vi "Ribbon Page.vi"() -> ()   [LabVIEW 2020, in "3D Ribbon.lvclass"]
uses:
  <vilib>/Math Plots/3D Math Plots/3D Ribbon/3D Ribbon/3D Ribbon.lvclass
  <vilib>/Math Plots/3D Math Plots/3D Ribbon/3D Ribbon/Typedef/3D Ribbon Property Array.ctl
  <vilib>/Math Plots/3D Math Plots/3D Ribbon/3D Ribbon/Typedef/3D Ribbon Property.ctl
  <vilib>/Math Plots/3D Math Plots/3D Plot/3D Plot/Typedef/Color Ramp Cluster.ctl
  <vilib>/Math Plots/3D Math Plots/3D Plot/3D Plot/Typedef/Line Type.ctl
  <vilib>/Math Plots/3D Math Plots/3D Plot/3D Plot/Typedef/Dialog State.ctl
  <vilib>/Math Plots/3D Math Plots/3D Plot/3D Plot/Typedef/Temp Scene State.ctl
  <vilib>/Math Plots/3D Math Plots/3D Plot/3D Plot/Typedef/Temp Scene Property Action.ctl
  <vilib>/Math Plots/3D Math Plots/3D Plot/3D Plot/3D Plot.lvclass
panel:
  in  "Ribbon Width":sgl=0.001 caption="Ribbon width" min=0.001 max=10 step=0.1
  in  "Ribbon Mode":u16(ring) caption="Ribbon mode" items=["Row", "Column"]
  in  "Draw Ribbon":bool caption="Draw ribbon"
  in  "Line Style":u16(ring) caption="Line style"
  in  "Antialiasing":bool
  in  "Line Width":sgl caption="Line width" min=0.001 step=1
  in  "Line Color":u32(colorbox) caption="Line color"
  out "Ribbon Property Out":T1
  in  "Ribbon Property In":T1
  out "Color Ramp":dbl[][](graph)
  in  "Color Map Style":u16(ring) caption="Color map style" items=["None ", "Shaded", "Color spectrum", "Grey scale", "Custom"]
  in  "YZ Plane Projection":bool caption="YZ  plane projection"
  in  "XZ Plane Projection":bool caption="XZ  plane projection"
  in  "XY Plane Projection":bool caption="XY plane projection"
  in  "Coordinate System":u16(ring) caption="Coordinate system" items=["Cartesian", "Cylindrical", "Spherical"]
  in  "Plot Opacity":sgl(slide) caption="Plot opacity(%)" min=0 max=100 scale=0.0..100.0
  in  "Plot List":i32(listbox)
  in  "Ramp Edit":bool caption="Ramp edit"
  in  "Move Down":bool
  in  "Move Up":bool
  in  "Delete":bool
  in  "New":bool
  in  "Event Registration":refnum<event-registration>
  # "Ribbon"
  # "General"
  # "Projection"
  # "Color Ramp"
  # "Ribbon"
  # "Outline"
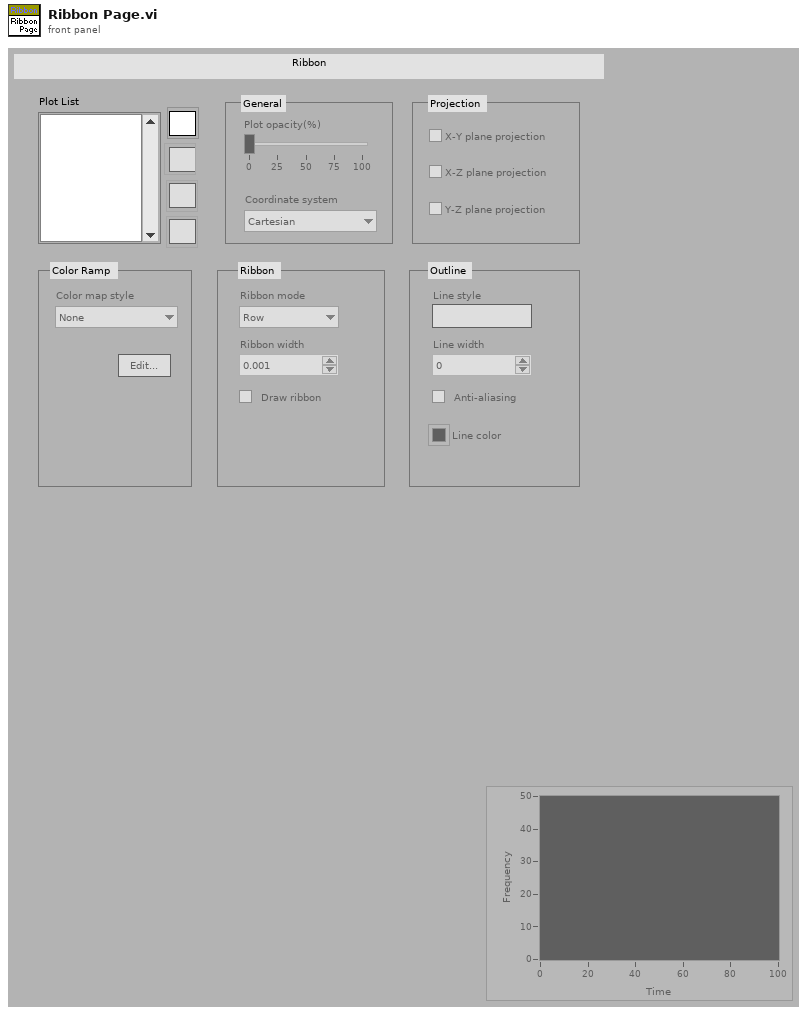
[diagram p1: front panel]
types:
  T1 = typedef "3D Ribbon.lvclass/3D Ribbon Property Array.ctl" = T2[]
  T2 = typedef "3D Ribbon.lvclass/3D Ribbon Property.ctl" = cluster{"General Property":cluster{"Plot Name":string, "Coordinate System":enum16{"Cartesian", "Cylindrical", "Spherical"}, "Opacity":sgl}, "Projection Property":cluster{"Draw XY":bool, "Draw YZ":bool, "Draw XZ":bool}, "Plot Property":cluster{"Draw Surface":bool, "Color Ramp Cluster":T3, "Line Style":T4, "Line Width":sgl, "Line Color":u32, "Antialiasing":bool}, "Ribbon Property":cluster{"Ribbon Mode":enum16{"Row", "Column"}, "Ribbon Width":sgl}}
  T3 = typedef "3D Plot.lvclass/Color Ramp Cluster.ctl" = cluster{"Color Ramp Style":enum16{"None", "Shaded", "Color spectrum", "Grey scale", "Custom"}, "Color Ramp Array":u32[], "Color Ramp Index":i32[], "Interpolate?":bool, "Logarithm?":bool}
  T4 = typedef "3D Plot.lvclass/Line Type.ctl" = enum16{"None", "Solid", "Dash", "Dot", "Dash Dot"}
  T5 = typedef "3D Plot.lvclass/Dialog State.ctl" = enum16{"Initialize", "Read Porperty", "Write Property", "Idle", "Exit"}
  T6 = typedef "3D Plot.lvclass/Temp Scene State.ctl" = enum16{"Create", "Update Scene", "Get Plot Representation", "Destory"}
  T7 = typedef "3D Plot.lvclass/Temp Scene Property Action.ctl" = enum16{"Graph Property", "Light Property", "Axis Property", "Value Pair Property", "Format Property", "Cursor Property", "Plot Specific Property"}
  T8 = typedef "3D Plot.lvclass/Multiplot Representation.ctl" = cluster{"Plot Represention Array":T9[], "Max Range":T10}
  T9 = typedef "3D Plot.lvclass/Plot Representation.ctl" = cluster{"Plot ID":i32, "Plot Range":T10, "Mesh Data":T11, "Dimension":cluster{"X Dimension":i32, "Y Dimension":i32}, "Ramp Range":T10}
  T10 = typedef "3D Plot.lvclass/Range Clusters.ctl" = cluster{"X Range":cluster{"Max X":sgl, "Min X":sgl}, "Y Range":cluster{"Max Y":sgl, "Min Y":sgl}, "Z Range":cluster{"Max Z":sgl, "Min Z":sgl}}
  T11 = typedef "3D Plot.lvclass/Mesh Data.ctl" = cluster{"Index Array":u32[], "Vertex Array":cluster{"X":sgl, "Y":sgl, "Z":sgl}[], "Normal Array":cluster{"X":sgl, "Y":sgl, "Z":sgl}[], "Color Index Array":i32[]}
  T12 = enum16{"None", "Shaded", "Color spectrum", "Grey scale", "Custom"}
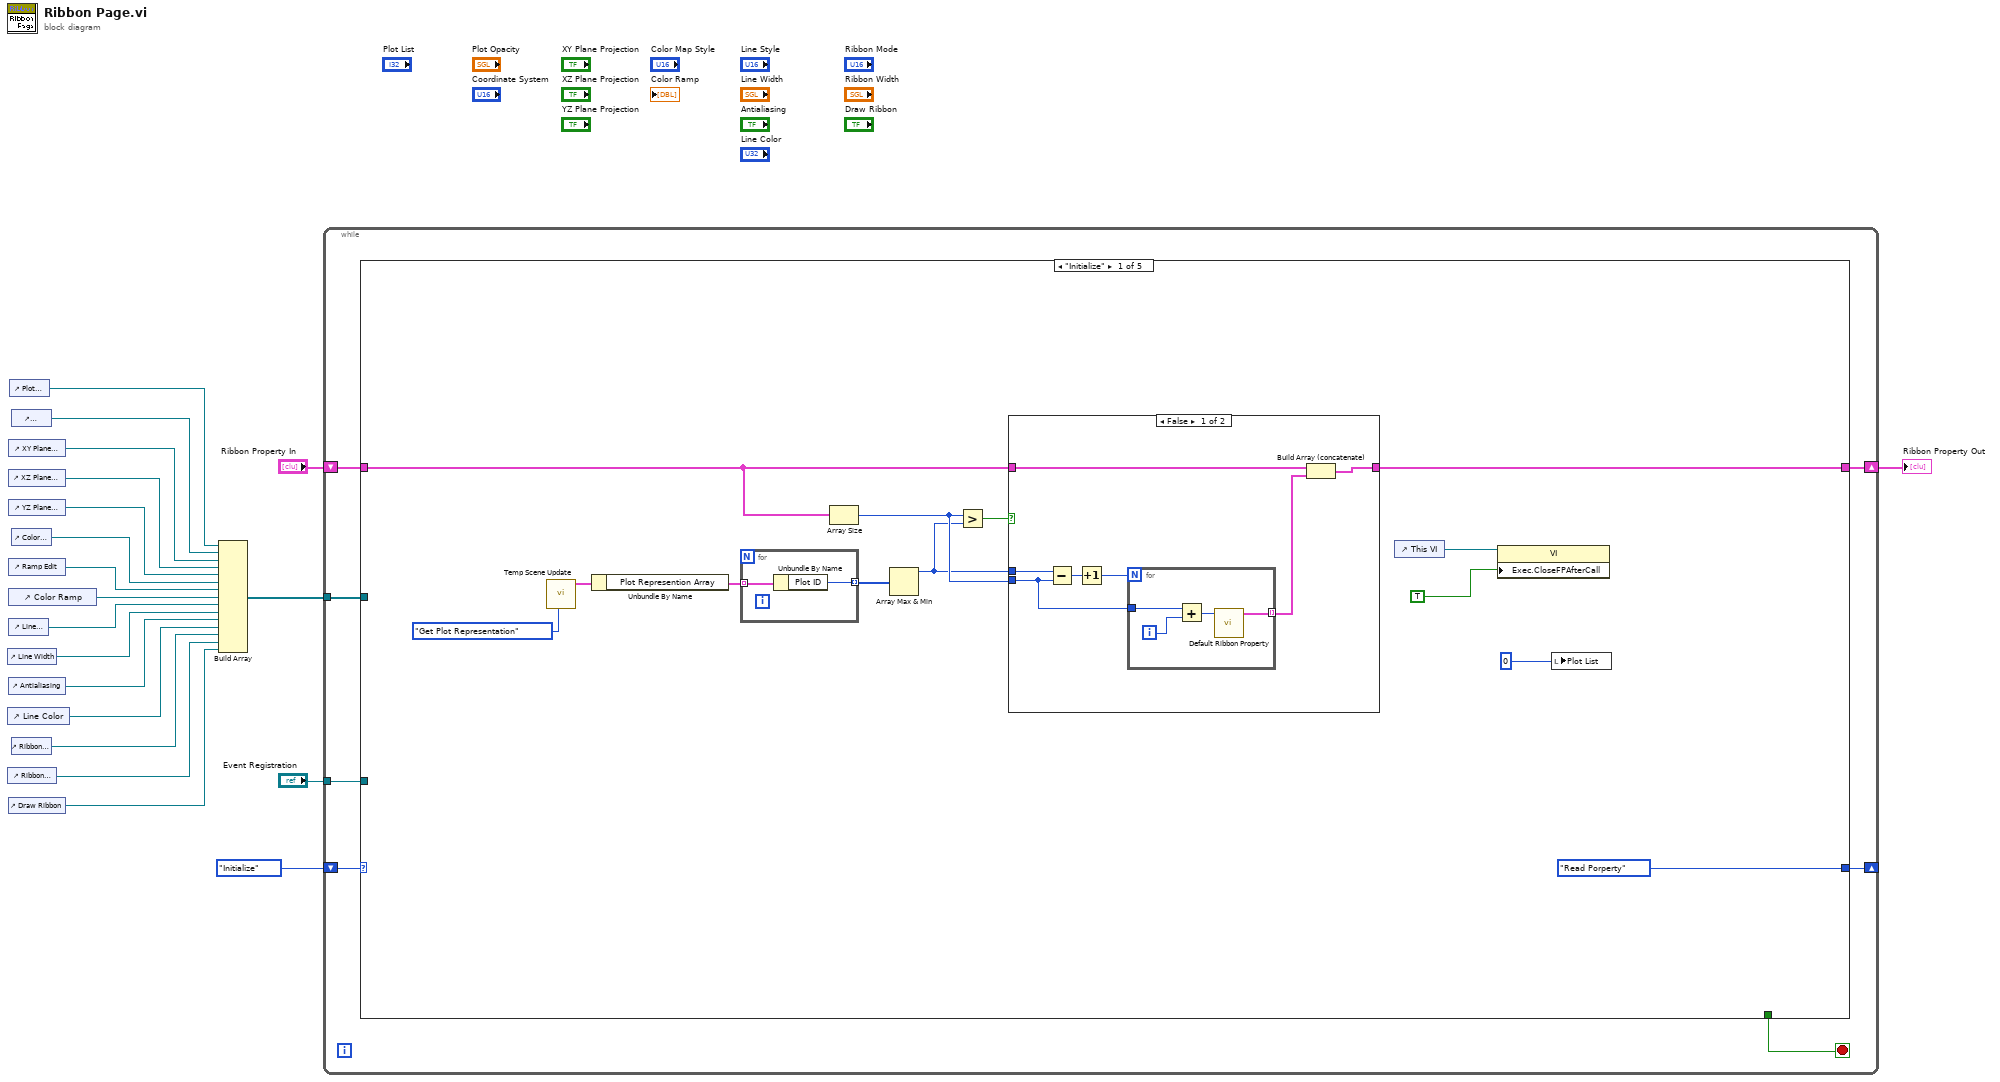
[diagram p0: block diagram]
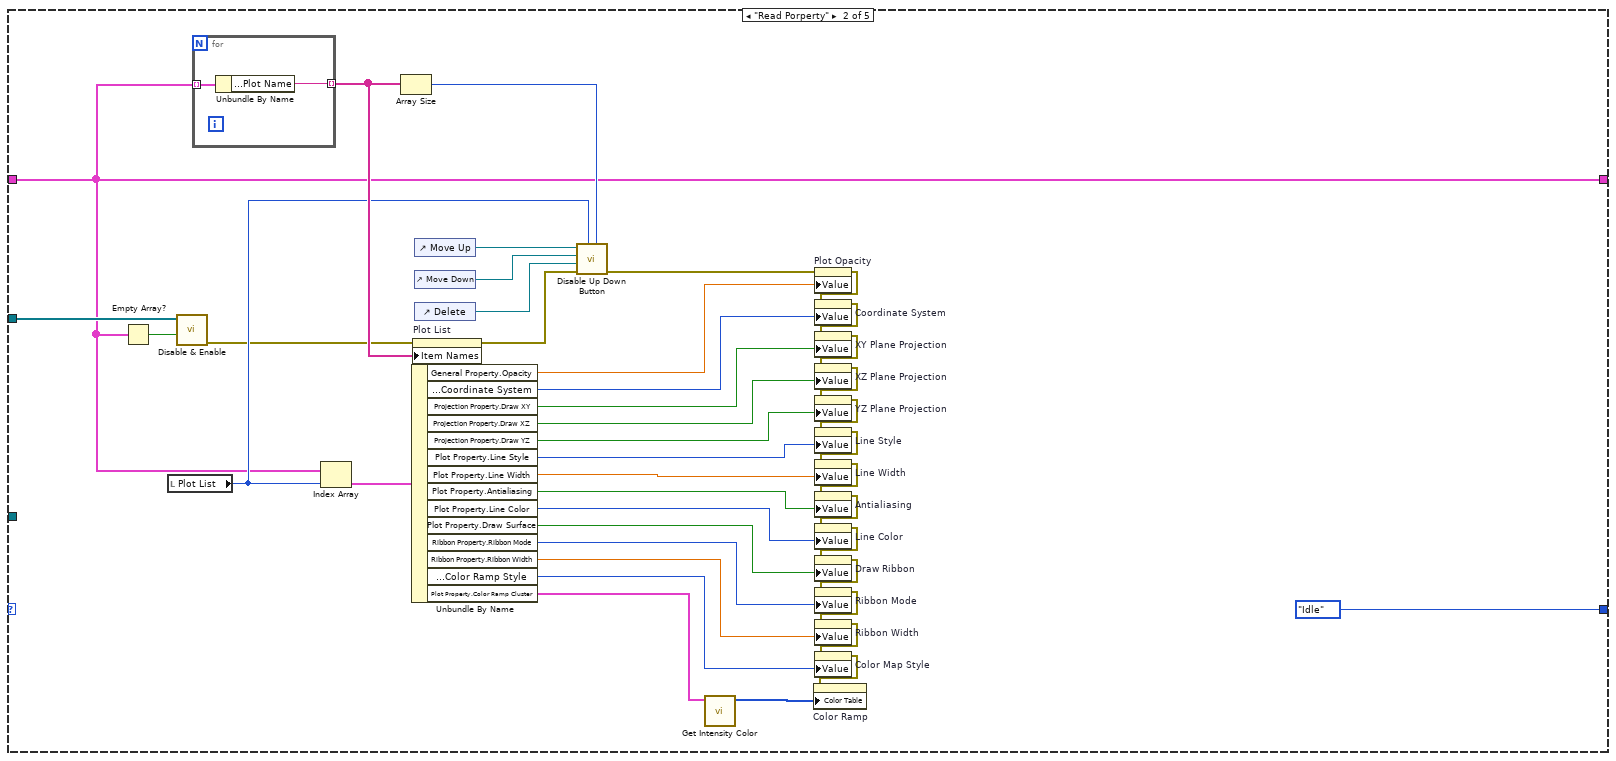
[diagram p3: hidden frame]
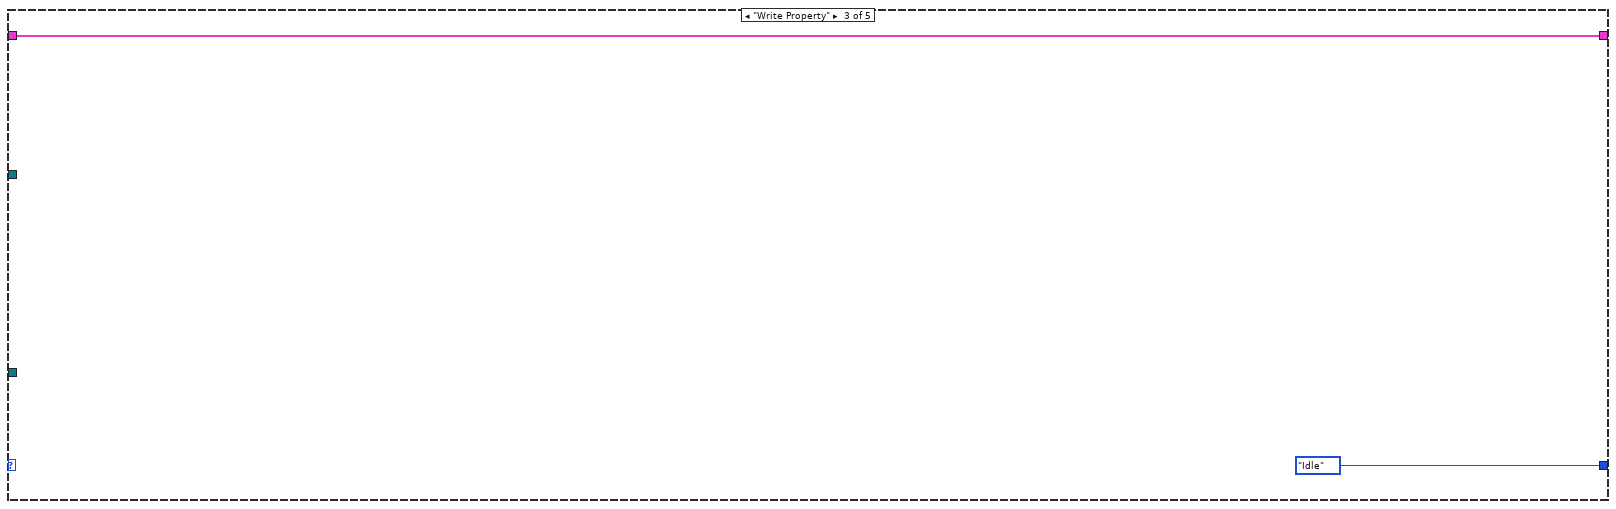
[diagram p4: hidden frame]
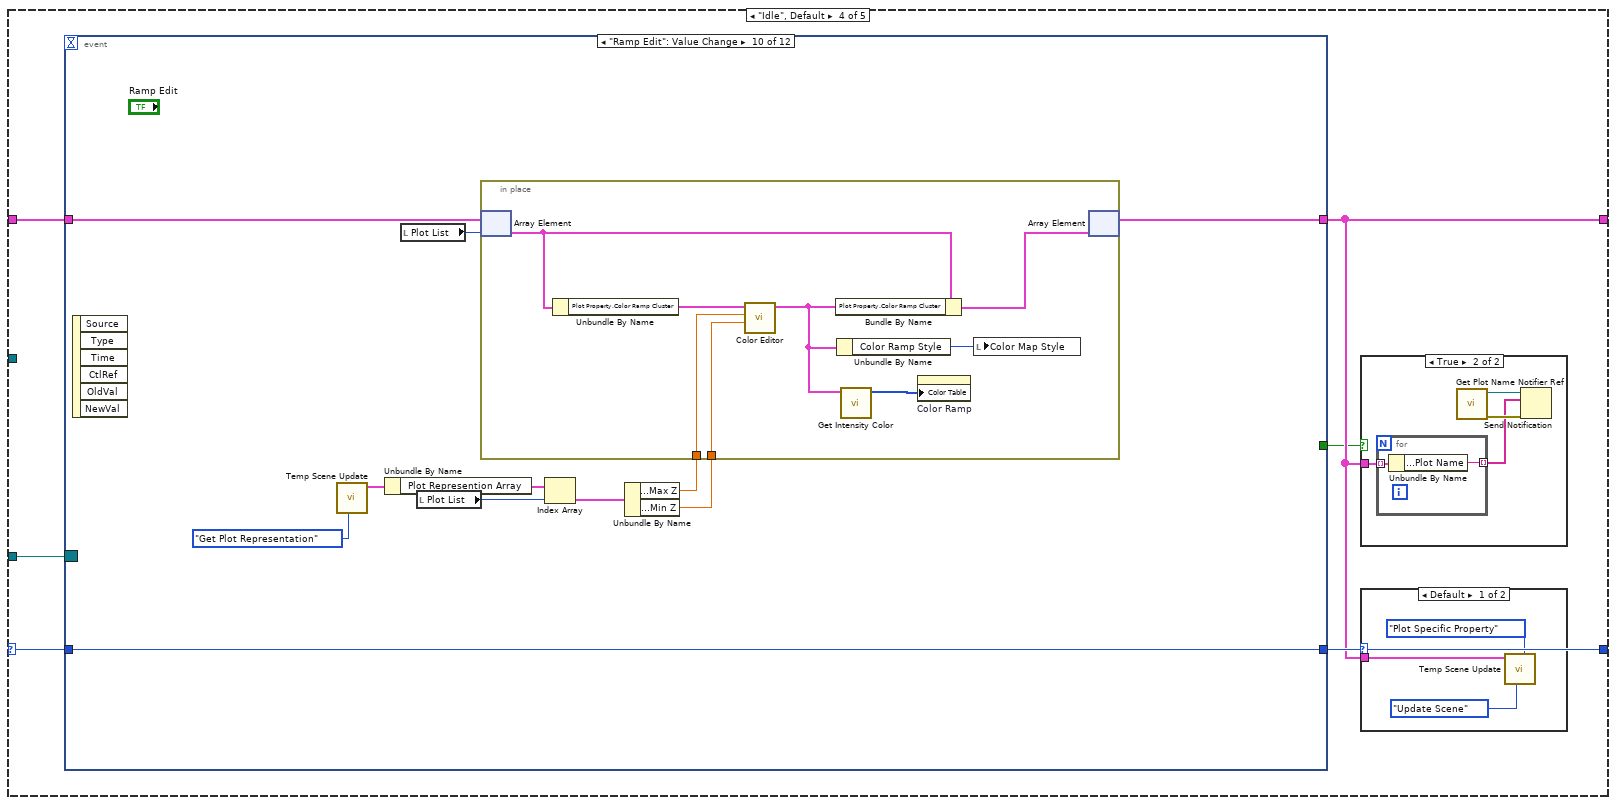
[diagram p5: hidden frame]
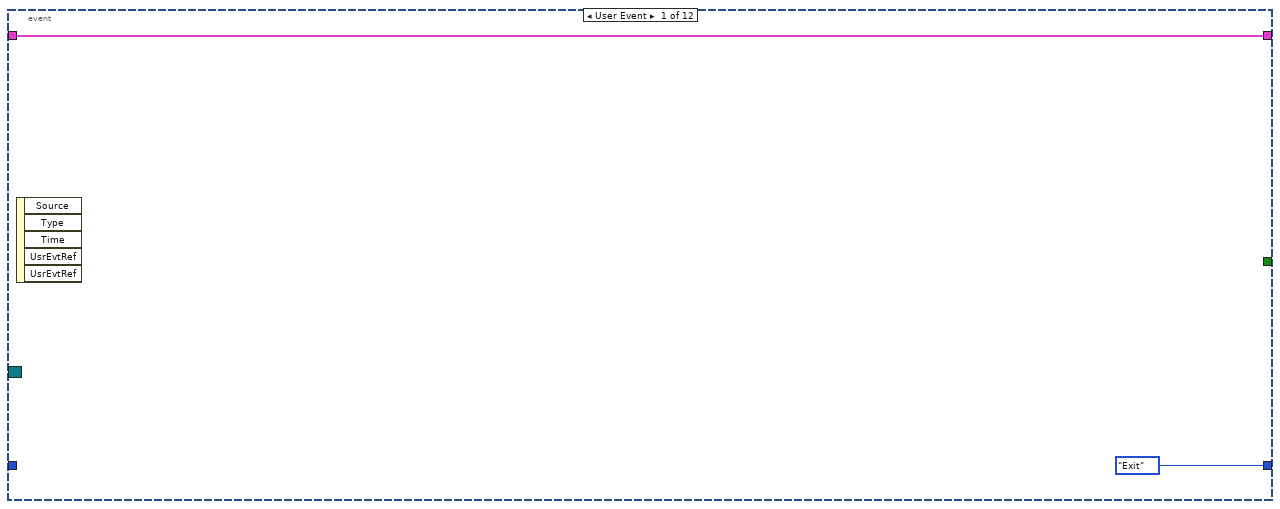
[diagram p8: hidden frame]
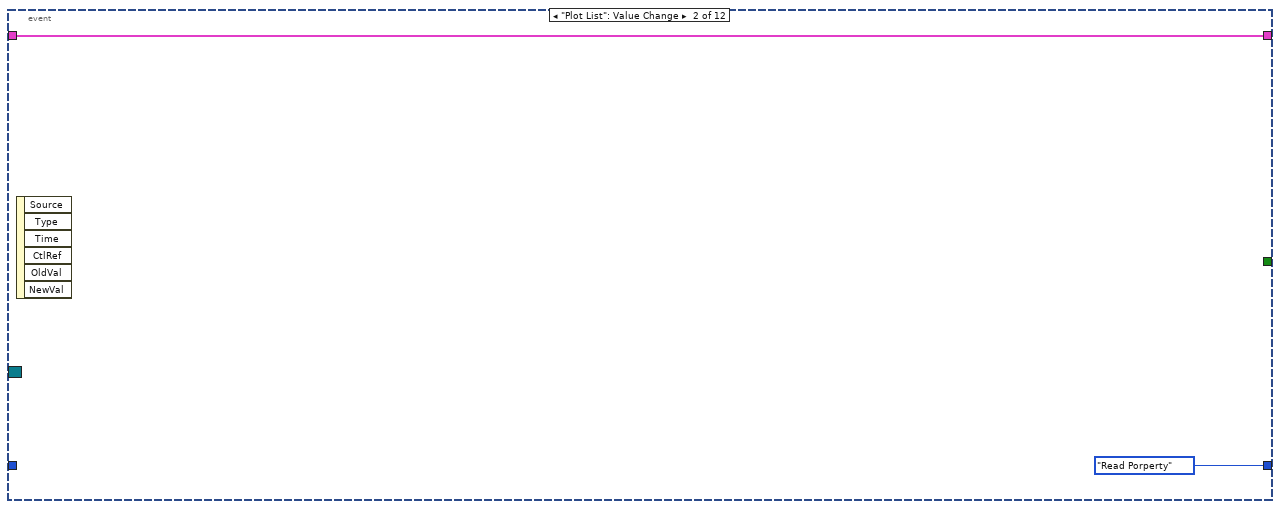
[diagram p9: hidden frame]
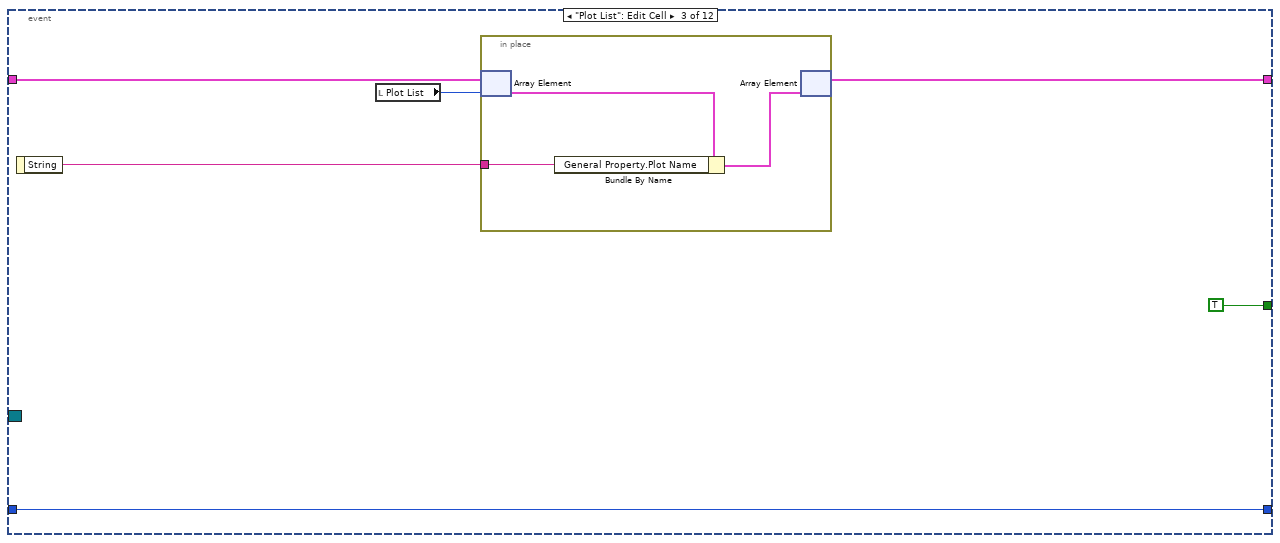
[diagram p10: hidden frame]
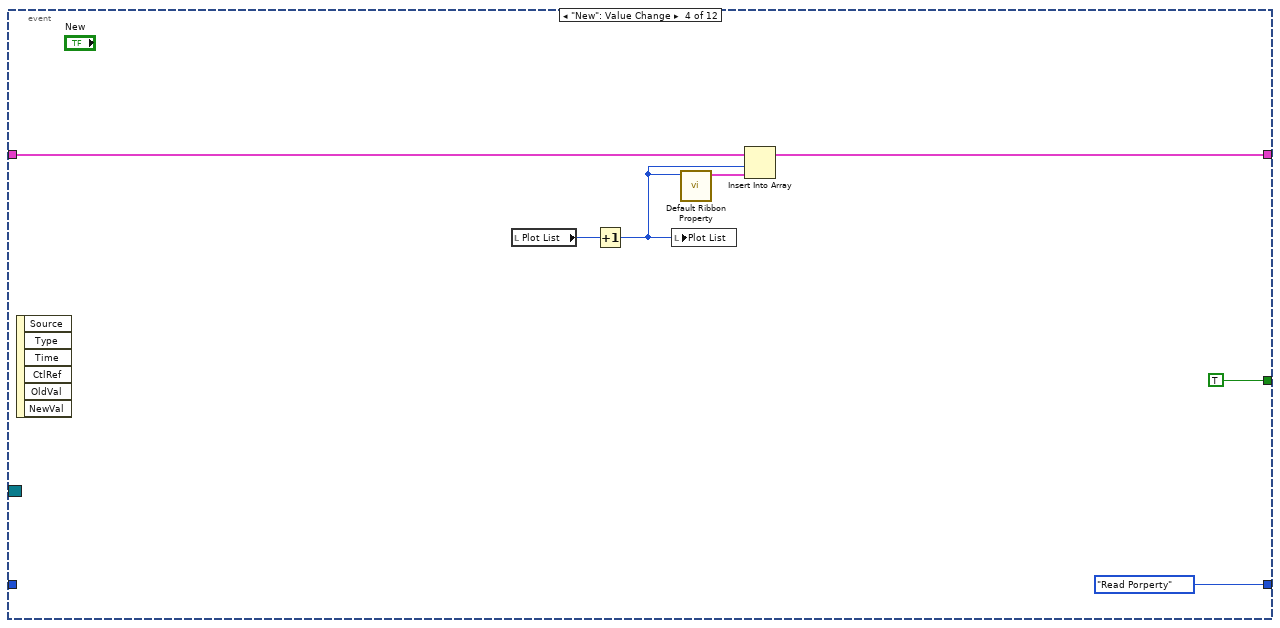
[diagram p11: hidden frame]
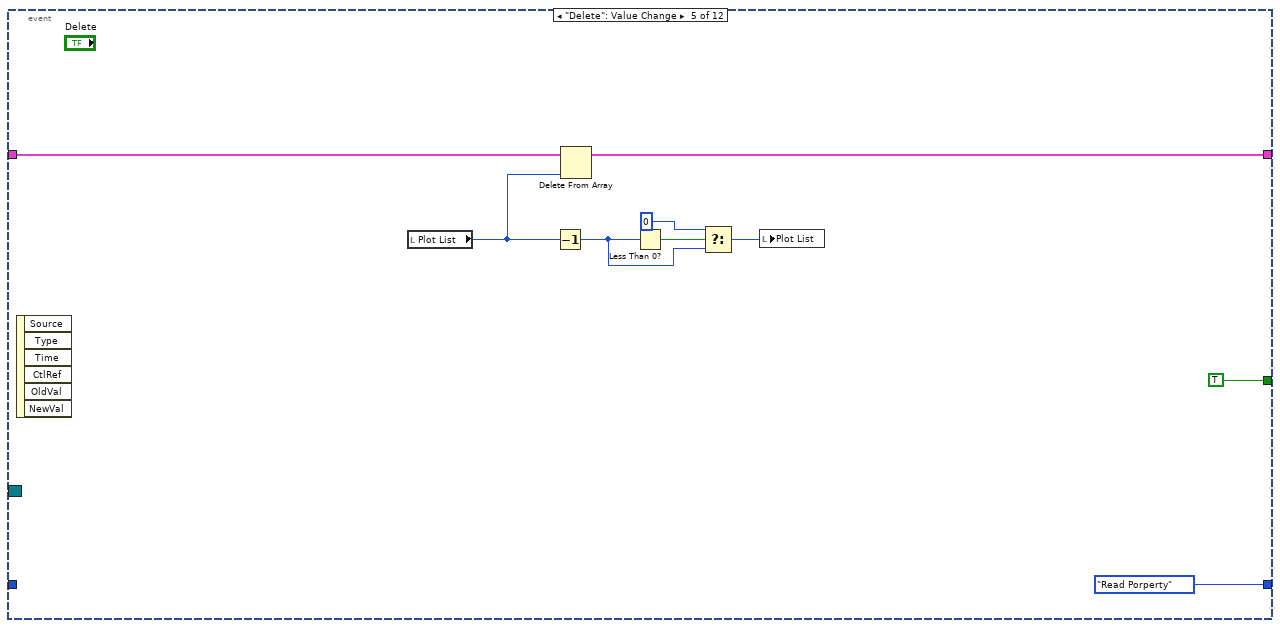
[diagram p12: hidden frame]
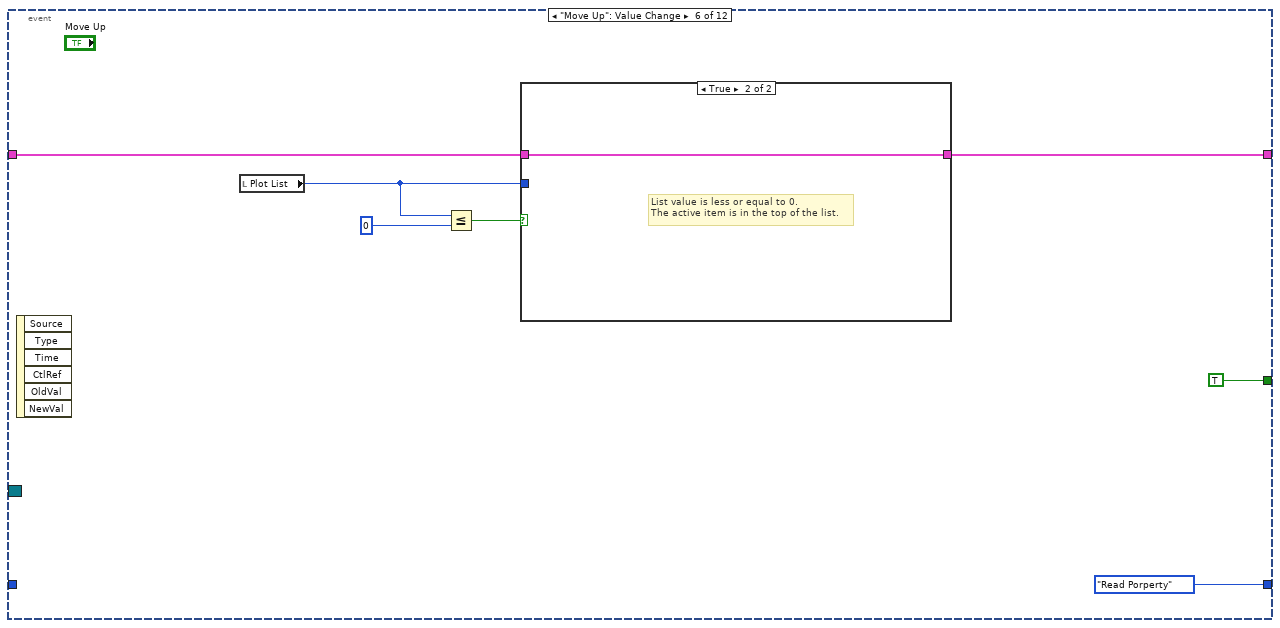
[diagram p13: hidden frame]
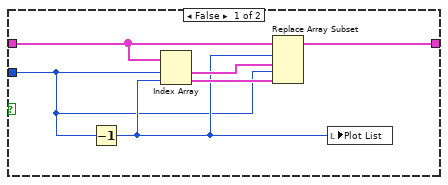
[diagram p14: hidden frame]
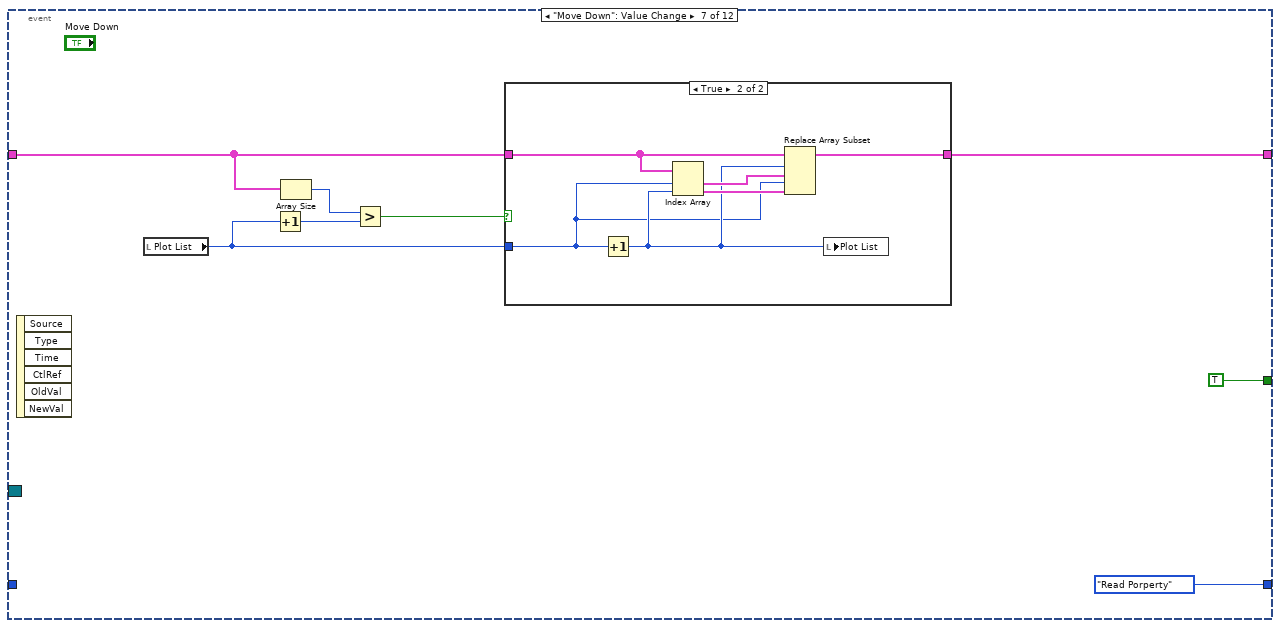
[diagram p15: hidden frame]
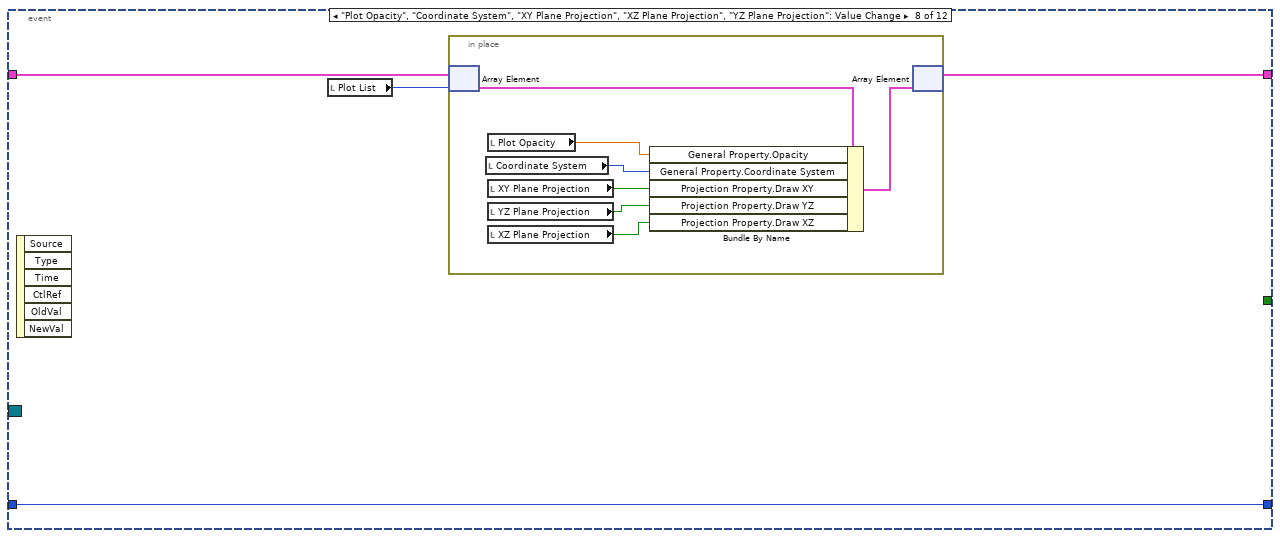
[diagram p17: hidden frame]
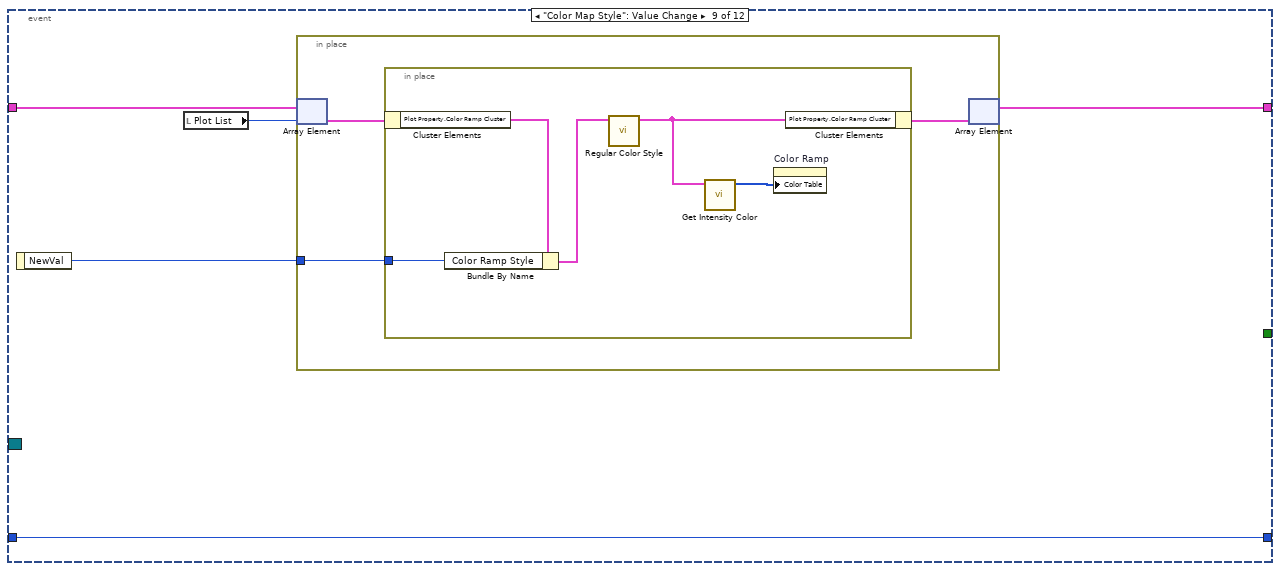
[diagram p18: hidden frame]
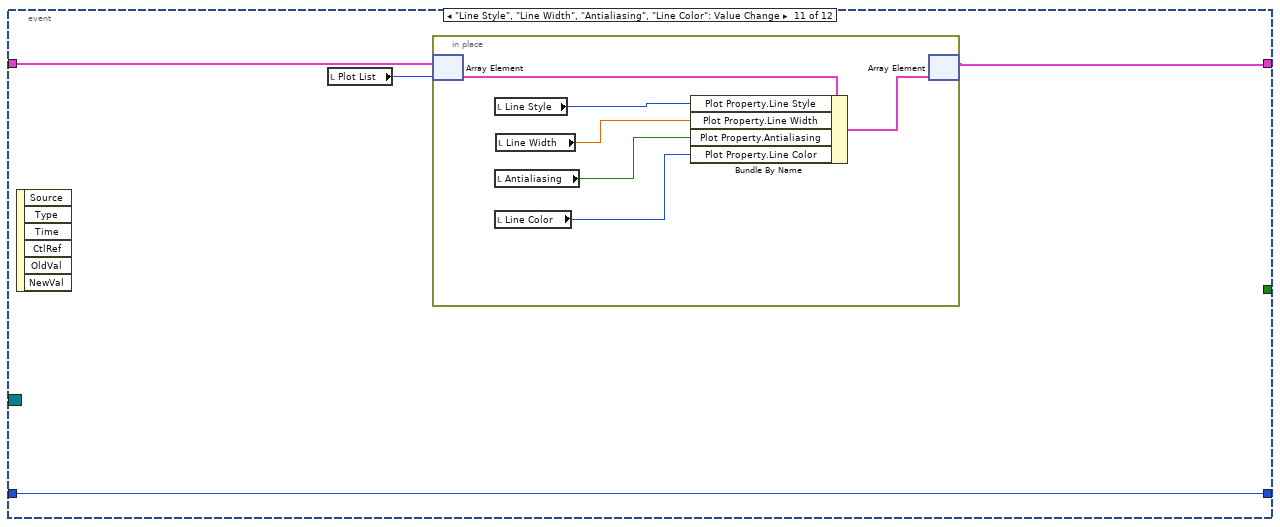
[diagram p19: hidden frame]
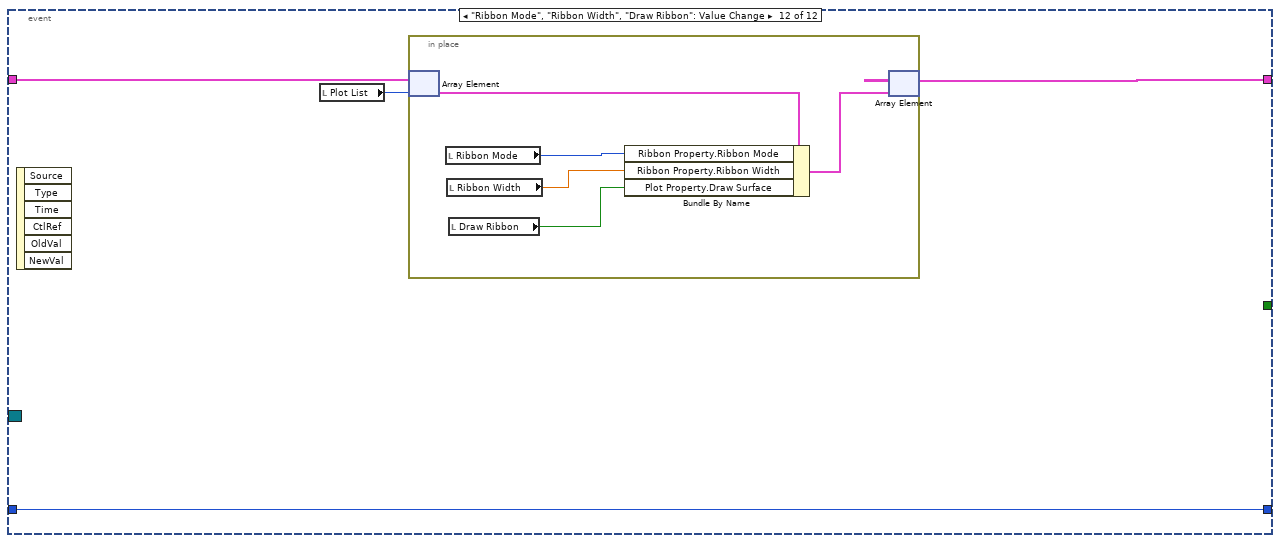
[diagram p20: hidden frame]
diagram:
  n1 = control-ref of="Line Width"() -> (w7:refnum<vi>)
  n2 = control-ref of="Line Color"() -> (w5:refnum<vi>)
  n3 = control-ref of="Ribbon Width"() -> (w3:refnum<vi>)
  n4 = control-ref of="XY Plane Projection"() -> (w14:refnum<vi>)
  n5 = control-ref of="XZ Plane Projection"() -> (w13:refnum<vi>)
  n6 = control-ref of="YZ Plane Projection"() -> (w12:refnum<vi>)
  n7 = control-ref of="Ramp Edit"() -> (w10:refnum<vi>)
  n8 = control-ref of="Color Ramp"() -> (w9:refnum<vi>)
  n9 = control-ref of="Line Style"() -> (w8:refnum<vi>)
  n10 = control-ref of="Antialiasing"() -> (w6:refnum<vi>)
  n11 = control-ref of="Draw Ribbon"() -> (w2:refnum<vi>)
  n12 = control-ref of="Plot Opacity"() -> (w16:refnum<vi>)
  n13 = control-ref of="Coordinate System"() -> (w15:refnum<vi>)
  n14 = control-ref of="Color Map Style"() -> (w11:refnum<vi>)
  n15 = control-ref of="Ribbon Mode"() -> (w4:refnum<vi>)
  n16 = Build Array(w16, w15, w14, w13, w12, w11, w10, w9, w8, w7, w6, w5, w4, w3, w2) -> (w1:refnum<vi>[])
  n17 = while {
    shift-right: [w26] -> w17
    shift-left: "Ribbon Property In" -> [w27]
    shift-right: [w22] -> _
    shift-left: Dialog_State."Initialize" -> [w25]
    tunnel: "Event Registration" -> [w23]
    tunnel: w1 -> [w21]
    stop <- w24 stop-if-true
    n18 = case shown="\"Initialize\"" w25 {
      selector: w25 -> [_ _ _ w104 _]
      tunnel: w27 -> [w30 w84 w99 w106 w236]
      tunnel: [w29 w84 w99 w102 w236] -> w26
      tunnel: [Dialog_State."Read Porperty" Dialog_State."Idle" Dialog_State."Idle" w103 Dialog_State."Exit"] -> w22
      tunnel: [_ _ _ _ TRUE] -> w24
      tunnel: w23 -> [_ _ _ w105 _]
      tunnel: w21 -> [_ w85 _ _ _]
      frame "Initialize" {
        n19 = call <vilib>:"Temp Scene Update.vi"("State"=Temp_Scene_State."Get Plot Representation") -> ("Multiplot Representation"=w35:T8)  [unwired: 5 in, 5 out]
        n20 = Unbundle By Name(w35) -> ("Plot Represention Array"=w28:T9[])
        n21 = for {
          tunnel: w28 -> [w54] mode=indexing
          tunnel: [w53] -> w34 mode=indexing
          n22 = Unbundle By Name(w54) -> ("Plot ID"=w53:i32)
        }
        n23 = Array Size(array=w30) -> (size(s)=w32:i32)
        n24 = Array Max & Min(array=w34) -> (max value=w31:i32)  [unwired: 3 out]
        n25 = Greater?(x=w32, y=w31) -> (0:w33:bool)
        n26 = case shown="False" w33 {
          tunnel: [w45 w52] -> w29
          tunnel: w30 -> [w47 w52]
          tunnel: w32 -> [w41 _]
          tunnel: w31 -> [w42 _]
          frame False {
            n27 = Subtract(x=w42, y=w41) -> (x-y=w44:i32)
            n28 = Increment(x=w44) -> (x+1=w43:i32)
            n29 = for {
              N: w43 -> [_]
              tunnel: w41 -> [w50]
              tunnel: [w48] -> w46 mode=indexing
              i -> [w51]
              n30 = Add(x=w50, y=w51) -> (x+y=w49:i32)
              n31 = call <vilib>:"Default Ribbon Property.vi"("Plot ID"=w49) -> ("Default Property"=w48:T2)  [unwired: 10 out]
            }
            n32 = Build Array (concatenate)(w47, w46) -> (w45:T1)
          }
          frame True {
          }
        }
        n33 = control-ref of="This VI"() -> (w39:refnum<vi>)
        n34 = property class="VI"(reference=w39, "Exec.CloseFPAfterCall"=TRUE ("Execution:Close After Call")) -> ()  [unwired: 1 in, 2 out]
        n35 = local write "Plot List"(0 ("Plot List")) -> ()
      }
      frame "Read Porperty" {
        n36 = Empty Array?(array=w84) -> (empty?=w86:bool)
        n37 = local read "Plot List"() -> (w87:i32)
        n38 = call <vilib>:"Disable & Enable.vi"("Disabled?"=w86, "Control Ref Array"=w85) -> ("error out"=w83:errorcluster)  [unwired: 1 in, 8 out]
        n39 = for {
          tunnel: w84 -> [w98] mode=indexing
          tunnel: [w97] -> w89 mode=indexing
          n40 = Unbundle By Name(w98) -> ("General Property.Plot Name"=w97:string)
        }
        n41 = Index Array(array=w84, index=w87) -> (element=w95:T2)
        n42 = Array Size(array=w89) -> (size(s)=w90:i32)
        n43 = Unbundle By Name(w95) -> ("General Property.Opacity"=w70:sgl, "General Property.Coordinate System"=w69:enum16{"Cartesian", "Cylindrical", "Spherical"}, "Projection Property.Draw XY"=w68:bool, "Projection Property.Draw XZ"=w67:bool, "Projection Property.Draw YZ"=w66:bool, "Plot Property.Line Style"=w65:T4, "Plot Property.Line Width"=w64:sgl, "Plot Property.Antialiasing"=w63:bool, "Plot Property.Line Color"=w62:u32, "Plot Property.Draw Surface"=w61:bool, "Ribbon Property.Ribbon Mode"=w60:enum16{"Row", "Column"}, "Ribbon Property.Ribbon Width"=w59:sgl, "Plot Property.Color Ramp Cluster.Color Ramp Style"=w58:T12, "Plot Property.Color Ramp Cluster"=w55:T3)
        n44 = property on="Plot List" class="LstBox (strict)"(error in=w83, "Item Names"=w89) -> (error out=w88:errorcluster)  [unwired: 1 in, 1 out]
        n45 = control-ref of="Move Up"() -> (w91:refnum<vi>)
        n46 = control-ref of="Move Down"() -> (w92:refnum<vi>)
        n47 = control-ref of="Delete"() -> (w93:refnum<vi>)
        n48 = call <vilib>:"Disable Up Down Button.vi"("Length"=w90, "Index"=w87, "error in (no error)"=w88, "Delete Ref"=w93, "Move Down Ref"=w92, "Move Up Ref"=w91) -> ("error out"=w57:errorcluster)  [unwired: 5 out]
        n49 = call <vilib>:"Get Intensity Color.vi"("Color Ramp Cluster"=w55) -> ("Intensity Color"=w94:u32[])  [unwired: 4 in, 6 out]
        n50 = property on="Plot Opacity" class="Slide (strict)"(error in=w57, "Value"=w70) -> (error out=w82:errorcluster)  [unwired: 1 in, 1 out]
        n51 = property on="Coordinate System" class="Ring (strict)"(error in=w82, "Value"=w69) -> (error out=w81:errorcluster)  [unwired: 1 in, 1 out]
        n52 = property on="XY Plane Projection" class="Bool (strict)"(error in=w81, "Value"=w68) -> (error out=w80:errorcluster)  [unwired: 1 in, 1 out]
        n53 = property on="XZ Plane Projection" class="Bool (strict)"(error in=w80, "Value"=w67) -> (error out=w79:errorcluster)  [unwired: 1 in, 1 out]
        n54 = property on="YZ Plane Projection" class="Bool (strict)"(error in=w79, "Value"=w66) -> (error out=w78:errorcluster)  [unwired: 1 in, 1 out]
        n55 = property on="Line Style" class="Ring (strict)"(error in=w78, "Value"=w65) -> (error out=w77:errorcluster)  [unwired: 1 in, 1 out]
        n56 = property on="Line Width" class="DigNum (strict)"(error in=w77, "Value"=w64) -> (error out=w76:errorcluster)  [unwired: 1 in, 1 out]
        n57 = property on="Antialiasing" class="Bool (strict)"(error in=w76, "Value"=w63) -> (error out=w75:errorcluster)  [unwired: 1 in, 1 out]
        n58 = property on="Line Color" class="ColBox"(error in=w75, "Value"=w62) -> (error out=w74:errorcluster)  [unwired: 1 in, 1 out]
        n59 = property on="Draw Ribbon" class="Bool (strict)"(error in=w74, "Value"=w61) -> (error out=w73:errorcluster)  [unwired: 1 in, 1 out]
        n60 = property on="Ribbon Mode" class="Ring (strict)"(error in=w73, "Value"=w60) -> (error out=w72:errorcluster)  [unwired: 1 in, 1 out]
        n61 = property on="Ribbon Width" class="DigNum (strict)"(error in=w72, "Value"=w59) -> (error out=w71:errorcluster)  [unwired: 1 in, 1 out]
        n62 = property on="Color Map Style" class="Ring (strict)"(error in=w71, "Value"=w58) -> (error out=w56:errorcluster)  [unwired: 1 in, 1 out]
        n63 = property on="Color Ramp" class="IntGraph (strict)"(error in=w56, "Color Table"=w94) -> ()  [unwired: 1 in, 2 out]
      }
      frame "Write Property" {
      }
      frame "Idle", Default {
        n64 = event shown="[9] \"Ramp Edit\": Value Change" {
          selector: w105 -> [_ _ _ _ _ _ _ _ _ _ _ _]
          dyn-events: _ -> [_ _ _ _ _ _ _ _ _ _ _ _]
          timeout: _ -> [_ _ _ _ _ _ _ _ _ _ _ _]
          tunnel: w106 -> [w117 w119 w123 w133 w142 w151 w161 w175 w188 w206 w218 w228]
          tunnel: [w117 w119 w122 w132 w143 w150 w166 w174 w185 w205 w217 w227] -> w102
          tunnel: [Dialog_State."Exit" Dialog_State."Read Porperty" w121 Dialog_State."Read Porperty" Dialog_State."Read Porperty" Dialog_State."Read Porperty" Dialog_State."Read Porperty" w177 w189 w208 w220 w229] -> w103
          tunnel: w104 -> [_ _ w121 _ _ _ _ w177 w189 w208 w220 w229]
          tunnel: [_ _ TRUE TRUE TRUE TRUE TRUE _ _ _ _ _] -> w101
          event User Event {
            n65 = event-data() -> ()  [unwired: 6 out]
          }
          event "Plot List": Value Change {
            n66 = event-data() -> ()  [unwired: 7 out]
          }
          event "Plot List": Edit Cell {
            n67 = event-data() -> ("String"=w124:string)  [unwired: 1 out]
            n68 = local read "Plot List"() -> (w125:i32)
            n69 = in-place {
              in-place-border: w124 -> [w126]
              n70 = in-place-array #1(w123, w125) -> (w128:T2)
              n71 = Bundle By Name(cluster=w128, "General Property.Plot Name"=w126) -> (w127:T2)
              n72 = in-place-array #1(w127) -> (w122:T1)  [unwired: 1 out]
            }
          }
          event "New": Value Change {
            n73 = event-data() -> ()  [unwired: 7 out]
            n74 = local read "Plot List"() -> (w134:i32)
            n75 = Increment(x=w134) -> (x+1=w130:i32)
            n76 = local write "Plot List"(w130) -> ()
            n77 = call <vilib>:"Default Ribbon Property.vi"("Plot ID"=w130) -> ("Default Property"=w129:T2)  [unwired: 10 out]
            n78 = Insert Into Array(array=w133, index=w130, new element=w129) -> (w132:T1)
          }
          event "Delete": Value Change {
            n79 = event-data() -> ()  [unwired: 7 out]
            n80 = local read "Plot List"() -> (w138:i32)
            n81 = Decrement(x=w138) -> (x-1=w139:i32)
            n82 = Delete From Array(array=w142, index=w138) -> (array with subset deleted=w143:T1)  [unwired: 1 in, 1 out]
            n83 = Less Than 0?(x=w139) -> (x < 0?=w141:bool)
            n84 = Select(t=0, s=w141, f=w139) -> (s? t:f=w137:i32)
            n85 = local write "Plot List"(w137) -> ()
          }
          event "Move Up": Value Change {
            n86 = event-data() -> ()  [unwired: 7 out]
            n87 = local read "Plot List"() -> (w146:i32)
            n88 = Less Or Equal?(x=w146, y=0) -> (x <= y?=w147:bool)
            n89 = case shown="True" w147 {
              tunnel: w151 -> [w155 w158]
              tunnel: [w154 w158] -> w150
              tunnel: w146 -> [w152 _]
              frame False {
                n90 = Decrement(x=w152) -> (x-1=w153:i32)
                n91 = Index Array(array=w155, index #1=w152, index #2=w153) -> (element #1=w157:T2, element #2=w156:T2)
                n92 = Replace Array Subset(array=w155, new element #1=w157, index #1=w153, new element #2=w156, index #2=w152) -> (w154:T1)
                n93 = local write "Plot List"(w153) -> ()
              }
              frame True {
                # "List value is less or equal to 0.\nThe active item is in the top of the list."
              }
            }
          }
          event "Move Down": Value Change {
            n94 = event-data() -> ()  [unwired: 7 out]
            n95 = local read "Plot List"() -> (w160:i32)
            n96 = Increment(x=w160) -> (x+1=w164:i32)
            n97 = Array Size(array=w161) -> (size(s)=w163:i32)
            n98 = Greater?(x=w163, y=w164) -> (0:w162:bool)
            n99 = case shown="True" w162 {
              tunnel: w160 -> [_ w170]
              tunnel: w161 -> [w167 w169]
              tunnel: [w167 w168] -> w166
              frame False {
                # "List value +1 is not less array length.\nThe active item is in the buttom of the list."
              }
              frame True {
                n100 = Increment(x=w170) -> (x+1=w171:i32)
                n101 = Index Array(array=w169, index #1=w170, index #2=w171) -> (element #1=w173:T2, element #2=w172:T2)
                n102 = Replace Array Subset(array=w169, new element #1=w173, index #1=w171, new element #2=w172, index #2=w170) -> (w168:T1)
                n103 = local write "Plot List"(w171) -> ()
              }
            }
          }
          event "Plot Opacity", "Coordinate System", "XY Plane Projection", "XZ Plane Projection", "YZ Plane Projection": Value Change {
            n104 = event-data() -> ()  [unwired: 7 out]
            n105 = local read "Plot List"() -> (w176:i32)
            n106 = in-place {
              n107 = in-place-array #2(w175, w176) -> (w180:T2)
              n108 = local read "Coordinate System"() -> (w178:u16)
              n109 = local read "Plot Opacity"() -> (w184:sgl)
              n110 = local read "XY Plane Projection"() -> (w183:bool)
              n111 = local read "YZ Plane Projection"() -> (w181:bool)
              n112 = local read "XZ Plane Projection"() -> (w182:bool)
              n113 = Bundle By Name(cluster=w180, "General Property.Opacity"=w184, "General Property.Coordinate System"=w178, "Projection Property.Draw XY"=w183, "Projection Property.Draw YZ"=w181, "Projection Property.Draw XZ"=w182) -> (w179:T2)
              n114 = in-place-array #2(w179) -> (w174:T1)  [unwired: 1 out]
            }
          }
          event "Color Map Style": Value Change {
            n115 = event-data() -> ("NewVal"=w186:u16)  [unwired: 1 out]
            n116 = local read "Plot List"() -> (w187:i32)
            n117 = in-place {
              in-place-border: w186 -> [w191]
              n118 = in-place-array #3(w188, w187) -> (w192:T2)
              n119 = in-place {
                in-place-border: w191 -> [w196]
                n120 = in-place-cluster #4(w192) -> ("Plot Property.Color Ramp Cluster"=w197:T3)
                n121 = Bundle By Name(cluster=w197, "Color Ramp Style"=w196) -> (w195:T3)
                n122 = call <vilib>:"Regular Color Style.vi"("Color Ramp Cluster in"=w195) -> ("Color Ramp Cluster out"=w193:T3)  [unwired: 10 in]
                n123 = call <vilib>:"Get Intensity Color.vi"("Color Ramp Cluster"=w193) -> ("Intensity Color"=w194:u32[])  [unwired: 4 in, 6 out]
                n124 = property on="Color Ramp" class="IntGraph (strict)"("Color Table"=w194) -> ()  [unwired: 2 in, 2 out]
                n125 = in-place-cluster #4("Plot Property.Color Ramp Cluster"=w193) -> (w190:T2)
              }
              n126 = in-place-array #3(w190) -> (w185:T1)  [unwired: 1 out]
            }
          }
          event "Ramp Edit": Value Change {
            n127 = event-data() -> ()  [unwired: 7 out]
            n128 = call <vilib>:"Temp Scene Update.vi"("State"=Temp_Scene_State."Get Plot Representation") -> ("Multiplot Representation"=w201:T8)  [unwired: 5 in, 5 out]
            n129 = Unbundle By Name(w201) -> ("Plot Represention Array"=w198:T9[])
            n130 = local read "Plot List"() -> (w207:i32)
            n131 = local read "Plot List"() -> (w204:i32)
            n132 = Index Array(array=w198, index=w204) -> (element=w203:T9)
            n133 = Unbundle By Name(w203) -> ("Plot Range.Z Range.Max Z"=w200:sgl, "Plot Range.Z Range.Min Z"=w199:sgl)
            n134 = in-place {
              in-place-border: w200 -> [w210]
              in-place-border: w199 -> [w209]
              n135 = in-place-array #5(w206, w207) -> (w215:T2)
              n136 = Unbundle By Name(w215) -> ("Plot Property.Color Ramp Cluster"=w214:T3)
              n137 = call <vilib>:"Color Editor.vi"("Min"=w209, "Max"=w210, "Color Ramp Cluster in"=w214) -> ("Color Ramp Cluster out"=w212:T3)  [unwired: 3 in, 5 out]
              n138 = Bundle By Name(cluster=w215, "Plot Property.Color Ramp Cluster"=w212) -> (w216:T2)
              n139 = Unbundle By Name(w212) -> ("Color Ramp Style"=w211:T12)
              n140 = call <vilib>:"Get Intensity Color.vi"("Color Ramp Cluster"=w212) -> ("Intensity Color"=w213:u32[])  [unwired: 4 in, 6 out]
              n141 = property on="Color Ramp" class="IntGraph (strict)"("Color Table"=w213) -> ()  [unwired: 2 in, 2 out]
              n142 = local write "Color Map Style"(w211) -> ()
              n143 = in-place-array #5(w216) -> (w205:T1)  [unwired: 1 out]
            }
          }
          event "Line Style", "Line Width", "Antialiasing", "Line Color": Value Change {
            n144 = event-data() -> ()  [unwired: 7 out]
            n145 = local read "Plot List"() -> (w219:i32)
            n146 = in-place {
              n147 = in-place-array #6(w218, w219) -> (w223:T2)
              n148 = local read "Line Style"() -> (w226:u16)
              n149 = local read "Antialiasing"() -> (w224:bool)
              n150 = local read "Line Color"() -> (w221:u32)
              n151 = local read "Line Width"() -> (w225:sgl)
              n152 = Bundle By Name(cluster=w223, "Plot Property.Line Style"=w226, "Plot Property.Line Width"=w225, "Plot Property.Antialiasing"=w224, "Plot Property.Line Color"=w221) -> (w222:T2)
              n153 = in-place-array #6(w222) -> (w217:T1)  [unwired: 1 out]
            }
          }
          event "Ribbon Mode", "Ribbon Width", "Draw Ribbon": Value Change {
            n154 = event-data() -> ()  [unwired: 7 out]
            n155 = local read "Plot List"() -> (w230:i32)
            n156 = in-place {
              n157 = in-place-array #7(w228, w230) -> (w235:T2)
              n158 = local read "Ribbon Mode"() -> (w232:u16)
              n159 = local read "Ribbon Width"() -> (w233:sgl)
              n160 = local read "Draw Ribbon"() -> (w231:bool)
              n161 = Bundle By Name(cluster=w235, "Ribbon Property.Ribbon Mode"=w232, "Ribbon Property.Ribbon Width"=w233, "Plot Property.Draw Surface"=w231) -> (w234:T2)
              n162 = in-place-array #7(w234) -> (w227:T1)  [unwired: 1 out]
            }
          }
        }
        n163 = case shown="True" w101 {
          tunnel: w102 -> [_ w107]
          frame False {
          }
          frame True {
            n164 = for {
              tunnel: w107 -> [w112] mode=indexing
              tunnel: [w111] -> w108 mode=indexing
              n165 = Unbundle By Name(w112) -> ("General Property.Plot Name"=w111:string)
            }
            n166 = call <vilib>:"Get Plot Name Notifier Ref.vi"() -> ("error out"=w110:errorcluster, "Plot Names Notifier Ref"=w109:refnum<notifier>)  [unwired: 1 in, 9 out]
            n167 = Send Notification(notification=w108, notifier=w109, error in (no error)=w110) -> ()  [unwired: 2 out]
          }
        }
        n168 = case shown="Default" w103 {
          tunnel: w102 -> [w115 _]
          frame Default {
            n169 = call <vilib>:"Temp Scene Update.vi"("Property Name"=Temp_Scene_Property_Action."Plot Specific Property", "State"=Temp_Scene_State."Update Scene", "Property In"=w115) -> ()  [unwired: 3 in, 6 out]
          }
          frame "Exit" {
          }
        }
      }
      frame "Exit" {
      }
    }
  }
  "Ribbon Property Out" <- w17
